vi "Scan_Hopping.vi"() -> ()   [LabVIEW 2023]
uses:
  Sub_Vi/TypeDefsControls/Xposition.ctl
  Sub_Vi/TypeDefsControls/Yposition.ctl
  Sub_Vi/TypeDefsControls/Piezo Velocity.ctl
  Sub_Vi/TypeDefsControls/Voltage.ctl
  Sub_Vi/TypeDefsControls/Zposition.ctl
  Sub_Vi/TypeDefs/Settings.ctl
  Sub_Vi/TypeDefs/ChangeOnFly.ctl
  Sub_Vi/TypeDefs/Display.ctl
  Sub_Vi/TypeDefsControls/Feedback Type.ctl
  Settings.vi
panel:
  in  "Feedback Type":T1
  in  "Retract Voltage (V)":T2=1.0 min=-10.0 max=10.0
  out "Estimated Time (mins)":dbl
  in  "Display Cluster":T3
  in  "ChangeonFly":T4
  in  "SettingsCluster":T5={"Sample Rate (us)"=1, "Samples Per Data Point (int, power of 2)"=1000, "DistanceToBulk (um)"=-1.0, "HoldTimeScaler"=1, "SaveData"=TRUE, "DistanceToBulk (um) 2"=-1.0, "DistanceToBulk (um) 3"=-1.0}
  in  "Retract after approach over":bool=TRUE
  in  "Greater Than":bool=TRUE
  in  "Hopping Approach Rate (µm/s)":T6=1.0 min=0.0
  in  "Hopping Retract Rate (µm/s)":T6=1.0 min=0.0
  in  "Hopping Distance (µm)":T7=1.0 min=0.0 max=100000.0
  in  "End Extension (µm)":T8=38.0 min=0.0 max=100000.0
  in  "ABSOLUTE Distance \nTo Retract (µm)":T8=1.0 min=0.0 max=100000.0
  in  "Upper dZ limit":i32=8
  in  "Feedback Threshold (A)":dbl=1e-13
  in  "P":fxp<+/-,32,1>=0.029999999795109034 format="%.32g"
  in  "X Center (µm)":T7=150.0 min=0.0 max=100000.0
  in  "Y Center (µm)":T9=150.0 min=0.0 max=100000.0
  in  "Y Width (µm)":T9=10.0 min=0.0 max=100000.0
  in  "X Width (µm)":T7=10.0 min=0.0 max=100000.0
  in  "Lateral Scan Rate (µm/s)":T6=1.0 min=0.0
  in  "Approach Voltage (V)":T2=1.0 min=-10.0 max=10.0
  in  "Approach Velocity (µm/s)":T6=1.0 min=0.0
  in  "Start Extension (µm)":T8 min=0.0 max=100000.0
  in  "Start scan Button":bool
  in  "Stop":bool
  in  "Pause":bool
  in  "Start Scanning Button":bool
  out "Y end":dbl
  out "X end":dbl
  out "X start":dbl
  out "Y start":dbl
  in  "Tab Control 4":T10(tab)=enum."Current Follower 3"
  out "Topography":dbl[][](graph)
  out "Current 1":dbl[][](graph)
  out "Current 2":dbl[][](graph)
  out "Current 3":dbl[][](graph)
  out "Z vs C3":cluster{"Y":dbl[], "Y":dbl[]}[](graph)
  out "Z vs C2":cluster{"Y":dbl[], "Y":dbl[]}[](graph)
  out "Lock In Phase":dbl[](graph)
  out "Lock In Amplitude":dbl[](graph)
  out "Z vs C1":cluster{"Y":dbl[], "Y":dbl[]}[](graph)
  out "t vs C3":dbl[](graph)
  out "t vs C2":dbl[](graph)
  out "t vs C1":dbl[](graph)
  # "Approach Settings"
  # "Pause at"
  # "Scan Settings"
  # "Define Scan Area"
  # "Change top/bottom values \ndepending on scan"
  # "Change top/bottom values \ndepending on scan"
  # "Change top/bottom values \ndepending on scan"
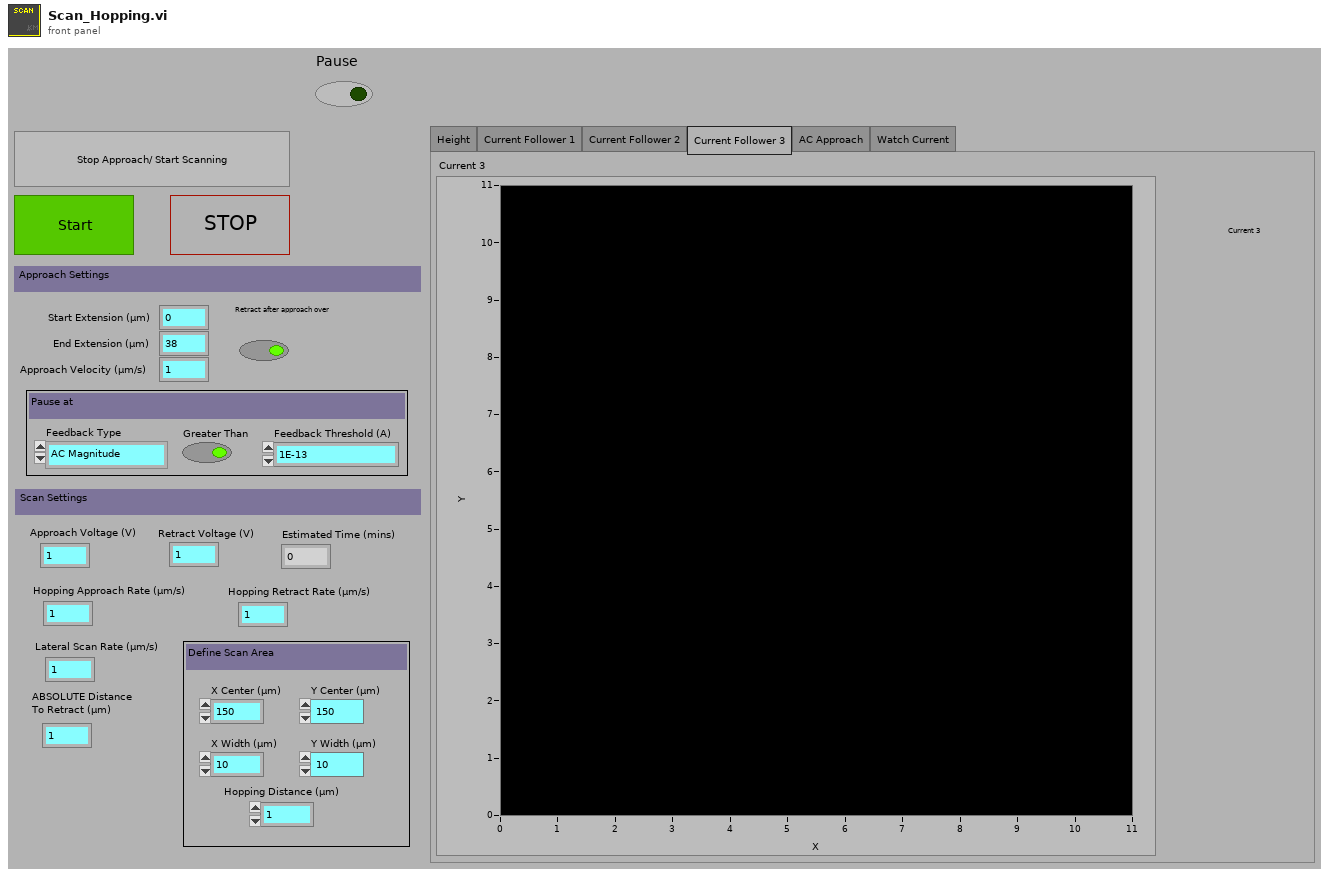
[diagram p1: front panel]
types:
  T1 = typedef "Feedback Type.ctl" = enum16{"AC Magnitude", "Current 1", "Current 2", "Phase"}
  T2 = typedef "Voltage.ctl" = dbl
  T3 = typedef "Display.ctl" = cluster{"X":refnum<vi>, "Y":refnum<vi>, "Z":refnum<vi>, "Amp":refnum<vi>, "Phase":refnum<vi>, "t vs Z":refnum<vi>, "t vs C1":refnum<vi>, "t vs C2":refnum<vi>, "t vs C3":refnum<vi>, "t vs Amp":refnum<vi>, "t vs Phase":refnum<vi>, "t vs X":refnum<vi>, "t vs Y":refnum<vi>, "Z vs C1":refnum<vi>, "Z vs C2":refnum<vi>, "Z vs C3":refnum<vi>, "V vs C1":refnum<vi>, "V vs C2":refnum<vi>, "V vs C3":refnum<vi>, "X/Y/Z F":refnum<vi>, "X/Y/Z R":refnum<vi>, "X/Y/C1 F":refnum<vi>, "X/Y/C1 R":refnum<vi>, "X/Y/C2 F":refnum<vi>, "X/Y/C2 R":refnum<vi>, "X/Y/C3 F":refnum<vi>, "X/Y/C3 R":refnum<vi>, "NumberOfLines":u16, "um Per Pixel":dbl, "um Per Line":dbl, "X Center":dbl, "Hop X/Y/Z":refnum<vi>, "Hop X/Y/C1":refnum<vi>, "Hop X/Y/C2":refnum<vi>, "Hop X/Y/C3":refnum<vi>, "X Width":dbl, "Y Width":dbl, "Hopping Distance":dbl, "V2 vs C1":refnum<vi>, "V vs Phase":refnum<vi>, "Y Center":dbl, "Number of Pixels":dbl, "V2 vs C2":refnum<vi>, "V2 vs C3":refnum<vi>, "V vs y":refnum<vi>, "V2 vs y":refnum<vi>, "Z vs Amp":refnum<vi>, "Z vs Phase":refnum<vi>}
  T4 = typedef "ChangeOnFly.ctl" = cluster{"Stop (boolean)":refnum<vi>, "Pause (boolean)":refnum<vi>, "EndCurrentLine (boolean)":refnum<vi>, "max movement per update step (Interger, nm)":refnum<vi>, "P (float, arb)":refnum<vi>, "Feedback set point (double, Amps)":refnum<vi>, "Voltage (double, V)":refnum<vi>, "Feedback set point 2 (double, Amps)":refnum<vi>, "Stop on Greater Than 2? (boolean)":refnum<vi>, "Stop on Greater Than? (boolean)":refnum<vi>, "Voltage 2 (double, V)":refnum<vi>, "Feedback Type (enum)":refnum<vi>, "Feedback Type 2 (enum)":refnum<vi>}
  T5 = typedef "Settings.ctl" = cluster{"Sample Rate (us)":u32, "Samples Per Data Point (int, power of 2)":i16, "DistanceToBulk (um)":dbl, "HoldTimeScaler":u64, "SaveData":bool, "DistanceToBulk (um) 2":dbl, "DistanceToBulk (um) 3":dbl}
  T6 = typedef "Piezo Velocity.ctl" = dbl
  T7 = typedef "Xposition.ctl" = dbl
  T8 = typedef "Zposition.ctl" = dbl
  T9 = typedef "Yposition.ctl" = dbl
  T10 = enum32{"Height", "Current Follower 1", "Current Follower 2", "Current Follower 3", "AC Approach", "Watch Current"}
  T11 = cluster{"Scan Rate (um/s)":dbl, "X Start":dbl, "X End":dbl, "Y Start":dbl, "Y End":dbl, " Z Start":dbl, "HoppingDistance":dbl, "V":dbl, "Z End":dbl, "Approach Rate Hopping (um/s)":dbl, "Retrack Rate (um/s)":dbl, "V 2":dbl, "Approach Rate (um/s)":dbl, "RetractV (V)":dbl}
  T12 = typedef "WayPointCluster.ctl" = cluster{"X (um)":dbl[], "Y (um)":dbl[], "Z (um)":dbl[], "V (V)":dbl[], "X Velocity (um s-1)":dbl[], "Y Velocity (um s-1)":dbl[], "Z Velocity (um s-1)":dbl[], "V Velocity (V s-1)":dbl[], "FeedBack Type (enum)":u16[], "Move X (boolean)":bool[], "Move Y (boolean)":bool[], "Move Z (boolean)":bool[], "Move V (boolean)":bool[], "Jump V (boolean)":bool[], "Hold (boolean)":bool[], "Hold Time":u32[], "V2 (V)":dbl[], "Move V2":bool[], "V2 Velocity (V s-1)":dbl[], "Jump V2 (boolean)":bool[], "Update z Position delta (ms)":i16[], "Hold Feedback1":bool[], "Move Z PicoMotor":bool[], " Z PicoMotor Direction":bool[], "DIO0":bool[]}
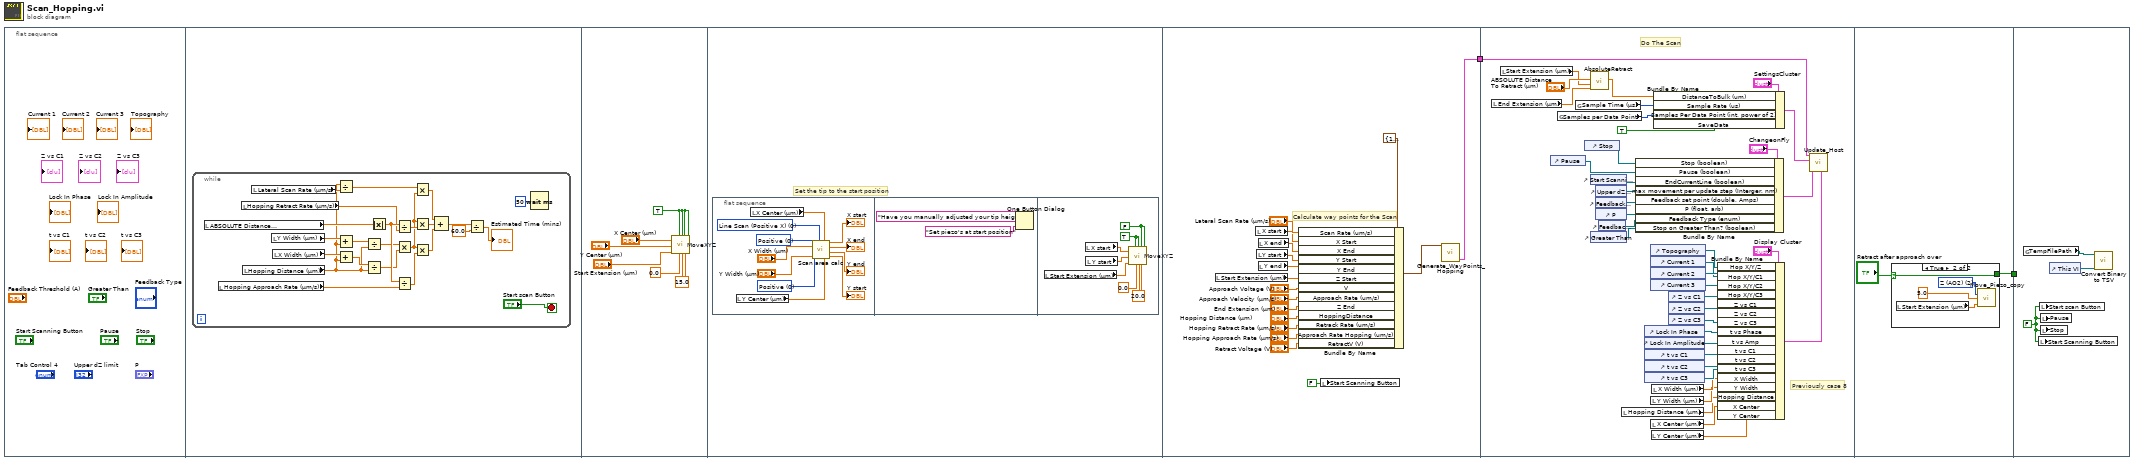
[diagram p0: block diagram]
diagram:
  n1 = flat-sequence {
    tunnel: [w66] -> w2
    tunnel: w2 -> [w108]
    tunnel: [w109] -> w1
    tunnel: w1 -> [_]
    frame #0 {
    }
    frame #1 {
      n2 = while {
        stop <- "Start scan Button" stop-if-true
        n3 = local read "ABSOLUTE Distance \nTo Retract (µm)"() -> (w13:T8)
        n4 = local read "Hopping Approach Rate (µm/s)"() -> (w6:T6)
        n5 = local read "Hopping Retract Rate (µm/s)"() -> (w4:T6)
        n6 = local read "Hopping Distance (µm)"() -> (w3:T7)
        n7 = local read "Lateral Scan Rate (µm/s)"() -> (w19:T6)
        n8 = local read "Y Width (µm)"() -> (w18:T9)
        n9 = local read "X Width (µm)"() -> (w17:T7)
        n10 = Divide(x=w3, y=w19) -> (x/y=w20:T7)
        n11 = Add(x=w18, y=w3) -> (x+y=w12:T9)
        n12 = Add(x=w17, y=w3) -> (x+y=w11:T7)
        n13 = Divide(x=w12, y=w3) -> (x/y=w9:T9)
        n14 = Divide(x=w11, y=w3) -> (x/y=w8:T7)
        n15 = Absolute Value(x=w13) -> (abs(x)=w14:T8)
        n16 = Divide(x=w14, y=w4) -> (x/y=w22:T8)
        n17 = Multiply(x=w9, y=w8) -> (x*y=w10:T9)
        n18 = Divide(x=w14, y=w6) -> (x/y=w15:T8)
        n19 = Multiply(x=w20, y=w10) -> (x*y=w21:T7)
        n20 = Multiply(x=w10, y=w22) -> (x*y=w5:T9)
        n21 = Multiply(x=w10, y=w15) -> (x*y=w16:T9)
        n22 = Compound Arithmetic op=ADD(w21, w5, w16) -> (w23:T7)
        n23 = Divide(x=w23, y=60.0) -> (x/y=→"Estimated Time (mins)":T7)
        n24 = Wait (ms)(milliseconds to wait=u32 50) -> ()  [unwired: 1 out]
      }
    }
    frame #2 {
      w31 = TRUE ("Set X")
      w32 = 15.0 ("Scan Rate (V/s) X and Y")
      n25 = call "MoveXYZ.vi"("X final height"="X Center (µm)", "Y final height"="Y Center (µm)", "Z final height"="Start Extension (µm)", "Set X"=w31, "V final"=0.0 ("Z initial height"), "Set Y"=w31, "Scan Rate (um/s)"=w32, "Set Z"=w31, "Scan Rate (V/s) 2"=w32, "Set Voltage"=w31) -> ()  [unwired: 10 in]
    }
    frame #3 {
      # "Set the tip to the start position"
      n26 = flat-sequence {
        frame #0 {
          w33 = u16 0 items=["Positive", "Negative"] ("Major Axis Direction")
          w34 = u16 0 items=["Positive", "Negative"] ("Minor Axis Direction")
          w35 = u16 0 items=["Line Scan (Positive X)", "Line Scan (Negative X)", "Line Scan (Positive Y)", "Line Scan (Negative Y)"] ("Scan Type")
          n27 = local read "Y Center (µm)"() -> (w36:T9)
          n28 = local read "X Center (µm)"() -> (w37:T7)
          n29 = call "Scan area calc.vi"("Y Width"="Y Width (µm)", "Major Axis Direction"=w33, "X Width"="X Width (µm)", "Minor Axis Direction"=w34, "Scan Type"=w35, "Y Center"=w36, "X Center"=w37) -> ("Y start"=→"Y start":dbl, "Y end"=→"Y end":dbl, "X end"=→"X end":dbl, "X start"=→"X start":dbl)
        }
        frame #1 {
          n30 = One Button Dialog(message="Have you manually adjusted your tip height", button name ("OK")="Set piezo's at start position") -> ()  [unwired: 1 out]
        }
        frame #2 {
          w48 = FALSE ("Set Z")
          w49 = TRUE ("Set X")
          w50 = 20.0 ("Scan Rate (V/s)")
          n31 = local read "Start Extension (µm)"() -> (w46:T8)
          n32 = local read "X start"() -> (w52:dbl)
          n33 = local read "Y start"() -> (w51:dbl)
          n34 = call "MoveXYZ.vi"("X final height"=w52, "Y final height"=w51, "Z final height"=w46, "Set X"=w49, "V final"=0.0 ("Scan Rate (V/s) X and Y"), "Set Y"=w49, "Scan Rate (um/s)"=w50, "Set Z"=w48, "Scan Rate (V/s) 2"=w50, "Set Voltage"=w48) -> ()  [unwired: 10 in]
        }
      }
    }
    frame #4 {
      # "Calculate way points for the Scan"
      n35 = local read "Start Extension (µm)"() -> (w60:T8)
      n36 = local read "X start"() -> (w64:dbl)
      n37 = local read "Y start"() -> (w62:dbl)
      n38 = local read "X end"() -> (w63:dbl)
      n39 = local read "Y end"() -> (w61:dbl)
      n40 = Bundle By Name(cluster=T11 {"Scan Rate (um/s)"=1.0, "X Start"=147.5, "X End"=152.5, "Y Start"=147.5, "Y End"=152.5, " Z Start"=0.0, "HoppingDistance"=2.0, "V"=1.0, "Z End"=38.0, "Approach Rate Hopping (um/s)"=1.0, "Retrack Rate (um/s)"=15.0, "V 2"=15.0, "Approach Rate (um/s)"=1.0, "RetractV (V)"=1.0} ("Input Cluster"), "Scan Rate (um/s)"="Lateral Scan Rate (µm/s)", "X Start"=w64, "X End"=w63, "Y Start"=w62, "Y End"=w61, "Z Start"=w60, "V"="Approach Voltage (V)", "Approach Rate (um/s)"="Approach Velocity (µm/s)", "Z End"="End Extension (µm)", "HoppingDistance"="Hopping Distance (µm)", "Retrack Rate (um/s)"="Hopping Retract Rate (µm/s)", "Approach Rate Hopping (um/s)"="Hopping Approach Rate (µm/s)", "RetractV (V)"="Retract Voltage (V)") -> (w67:T11)
      n41 = local write "Start Scanning Button"(FALSE ("Start Scanning Button")) -> ()
      n42 = call "Generate_WayPoints_Hopping.vi"("Input Cluster"=w67) -> ("output cluster"=w66:T12)  [unwired: 10 in]
    }
    frame #5 {
      # "Previously case 8"
      # "Do The Scan"
      n43 = local read "End Extension (µm)"() -> (w71:T8)
      n44 = local read "Start Extension (µm)"() -> (w72:T8)
      n45 = control-ref of="Pause"() -> (w100:refnum<vi>)
      n46 = global read "Settings.vi" "Samples per Data Point"() -> (w82:u16)
      n47 = global read "Settings.vi" "Sample Time (µs)"() -> (w87:u32)
      n48 = control-ref of="Stop"() -> (w86:refnum<vi>)
      n49 = call "AbsoluteRetract.vi"("Z End"=w71, "Z Start height"=w72, "Distance To Retract / um"="ABSOLUTE Distance \nTo Retract (µm)") -> ("Distance To Retract / um 2"=w73:dbl)  [unwired: 8 in]
      n50 = control-ref of="Start Scanning Button"() -> (w104:refnum<vi>)
      n51 = control-ref of="Greater Than"() -> (w85:refnum<vi>)
      n52 = control-ref of="Upper dZ limit"() -> (w103:refnum<vi>)
      n53 = control-ref of="Feedback Threshold (A)"() -> (w101:refnum<vi>)
      n54 = control-ref of="P"() -> (w102:refnum<vi>)
      n55 = control-ref of="Feedback Type"() -> (w84:refnum<vi>)
      n56 = local read "Hopping Distance (µm)"() -> (w78:T7)
      n57 = Bundle By Name(cluster="ChangeonFly", "Stop (boolean)"=w86, "Pause (boolean)"=w100, "EndCurrentLine (boolean)"=w104, "max movement per update step (Interger, nm)"=w103, "Feedback set point (double, Amps)"=w101, "P (float, arb)"=w102, "Feedback Type (enum)"=w84, "Stop on Greater Than? (boolean)"=w85) -> (w105:T4)
      n58 = control-ref of="Lock In Phase"() -> (w96:refnum<vi>)
      n59 = control-ref of="Lock In Amplitude"() -> (w97:refnum<vi>)
      n60 = control-ref of="t vs C1"() -> (w98:refnum<vi>)
      n61 = control-ref of="t vs C2"() -> (w99:refnum<vi>)
      n62 = control-ref of="t vs C3"() -> (w81:refnum<vi>)
      n63 = control-ref of="Topography"() -> (w91:refnum<vi>)
      n64 = control-ref of="Current 1"() -> (w75:refnum<vi>)
      n65 = control-ref of="Current 2"() -> (w92:refnum<vi>)
      n66 = control-ref of="Current 3"() -> (w93:refnum<vi>)
      n67 = local read "Y Width (µm)"() -> (w79:T9)
      n68 = local read "X Center (µm)"() -> (w77:T7)
      n69 = local read "Y Center (µm)"() -> (w76:T9)
      n70 = local read "X Width (µm)"() -> (w80:T7)
      n71 = Bundle By Name(cluster="SettingsCluster", "DistanceToBulk (um)"=w73, "Sample Rate (us)"=w87, "Samples Per Data Point (int, power of 2)"=w82, "SaveData"=TRUE) -> (w106:T5)
      n72 = control-ref of="Z vs C1"() -> (w94:refnum<vi>)
      n73 = control-ref of="Z vs C2"() -> (w95:refnum<vi>)
      n74 = control-ref of="Z vs C3"() -> (w83:refnum<vi>)
      n75 = Bundle By Name(cluster="Display Cluster", "Hop X/Y/Z"=w91, "Hop X/Y/C1"=w75, "Hop X/Y/C2"=w92, "Hop X/Y/C3"=w93, "Z vs C1"=w94, "Z vs C2"=w95, "Z vs C3"=w83, "t vs Phase"=w96, "t vs Amp"=w97, "t vs C1"=w98, "t vs C2"=w99, "t vs C3"=w81, "X Width"=w80, "Y Width"=w79, "Hopping Distance"=w78, "X Center"=w77, "Y Center"=w76) -> (w107:T3)
      n76 = call "Update_Host.vi"("Display Cluster"=w107, "ChangeonFly"=w105, "SettingsCluster"=w106, "WayPointCluster"=w108) -> ()  [unwired: 6 in]
    }
    frame #6 {
      n77 = case shown="True" "Retract after approach over" {
        selector: "Retract after approach over" -> [w111 w112]
        tunnel: [w111 w112] -> w109
        frame False {
        }
        frame True {
          w115 = u16 2 items=["X (AO0)", "Y (AO1)", "Z (AO2)", "V (AO3)"] ("Channel")
          n78 = local read "Start Extension (µm)"() -> (w113:T8)
          n79 = call "Move_Piezo_copy.vi"("Piezo"=w115, "Movement Speed (µm/s)"=5.0 ("Scan Rate (um/s)"), "Position (µm) (or V)"=w113) -> ()  [unwired: 13 in]
        }
      }
    }
    frame #7 {
      w118 = FALSE ("Stop")
      n80 = global read "Settings.vi" "TempFilePath"() -> (w116:path)
      n81 = local write "Start Scanning Button"(w118) -> ()
      n82 = local write "Start scan Button"(w118) -> ()
      n83 = local write "Pause"(w118) -> ()
      n84 = local write "Stop"(w118) -> ()
      n85 = control-ref of="This VI"() -> (w117:refnum<vi>)
      n86 = call "Convert Binary to TSV.vi"("This VI"=w117, "TDMS DataFile Name"=w116) -> ()  [unwired: 10 in]
    }
  }
